vi "Configure Glitch Trigger Source.vi"(0 "VISA resource name":refnum<visa-resource-name>, 5 "Trigger Source (0: Channel 1)":u16(ring) items=["Channel 1", "Channel 2", "Channel 3", "Channel 4", "DIG 0", "DIG 1", "DIG 2", "DIG 3", "DIG 4", "DIG 5", "DIG 6", "DIG 7", "DIG 8", "DIG 9", "DIG 10", "DIG 11", "DIG 12", "DIG 13", "DIG 14", "DIG 15", "External"], 7 "Trigger Level (0.0)":dbl, 9 "Glitch Condition (0: Less Than)":u16(ring) items=["Less Than", "Greater Than", "Range"], 11 "error in (no error)":errorcluster, 12 "Glitch Polarity (0: Positive)":u16(ring) items=["Positive", "Negative"], 13 "Maximum (2)":dbl=2.0, 14 "Minimum (1)":dbl=1.0) -> (4 "VISA resource name out":refnum<visa-resource-name>, 15 "error out":errorcluster)   [LabVIEW 2017, in "Agilent 6000 Series.lvlib"]
doc: "This VI configures the glitch trigger. You specify the condition with the Glitch Condition property and polarity of the pulse with the Glitch Polarity parameter. The trigger does not actually occur until the edge of a pulse that corresponds to the Glitch Width and Glitch Polarity crosses the threshold you specify in the Trigger Level parameter."
uses:
  <instrlib>/Agilent 6000 Series/Agilent 6000 Series.lvlib
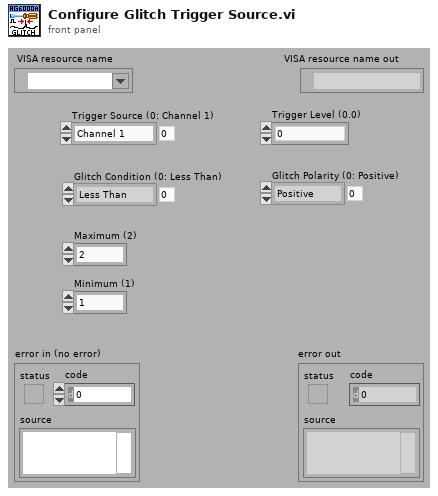
[diagram p1: front panel]
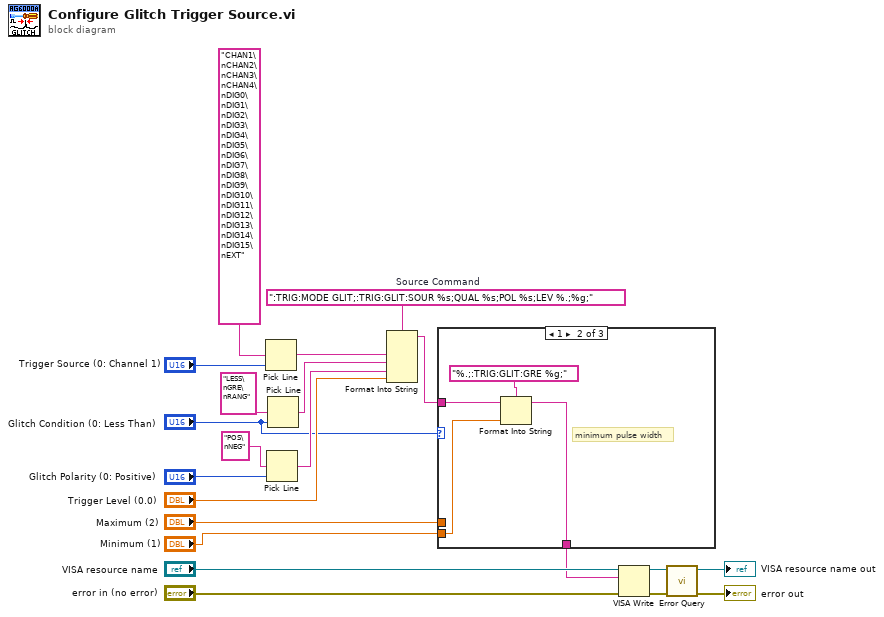
[diagram p0: block diagram]
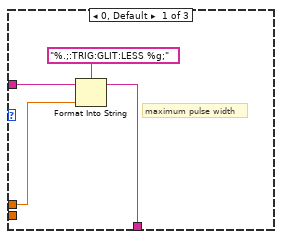
[diagram p2: hidden frame]
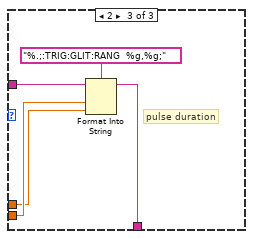
[diagram p3: hidden frame]
diagram:
  w15 = ":TRIG:MODE GLIT;:TRIG:GLIT:SOUR %s;QUAL %s;POL %s;LEV %.;%g;"  # Source Command
  n1 = Pick Line(multi-line string="CHAN1\nCHAN2\nCHAN3\nCHAN4\nDIG0\nDIG1\nDIG2\nDIG3\nDIG4\nDIG5\nDIG6\nDIG7\nDIG8\nDIG9\nDIG10\nDIG11\nDIG12\nDIG13\nDIG14\nDIG15\nEXT", line index="Trigger Source (0: Channel 1)") -> (output string=w14:string)  [unwired: 1 in]
  n2 = Pick Line(multi-line string="POS\nNEG", line index="Glitch Polarity (0: Positive)") -> (output string=w8:string)  [unwired: 1 in]
  n3 = Pick Line(multi-line string="LESS\nGRE\nRANG", line index="Glitch Condition (0: Less Than)") -> (output string=w11:string)  [unwired: 1 in]
  n4 = Format Into String(format string=w15, w14, w11, w8, "Trigger Level (0.0)") -> (resulting string=w4:string)  [unwired: 2 in, 1 out]
  n5 = case shown="1" "Glitch Condition (0: Less Than)" {
    tunnel: "Maximum (2)" -> [w24 _ w30]
    tunnel: w4 -> [w23 w28 w33]
    tunnel: [w22 w26 w31] -> w3
    tunnel: "Minimum (1)" -> [_ w27 w32]
    frame 0, Default {
      # "maximum pulse width"
      n6 = Format Into String(format string="%.;:TRIG:GLIT:LESS %g;", initial string=w23, w24) -> (resulting string=w22:string)  [unwired: 1 in, 1 out]
    }
    frame 1 {
      # "minimum pulse width"
      n7 = Format Into String(format string="%.;:TRIG:GLIT:GRE %g;", initial string=w28, w27) -> (resulting string=w26:string)  [unwired: 1 in, 1 out]
    }
    frame 2 {
      # "pulse duration"
      n8 = Format Into String(format string="%.;:TRIG:GLIT:RANG  %g,%g;", initial string=w33, w32, w30) -> (resulting string=w31:string)  [unwired: 1 in, 1 out]
    }
  }
  n9 = VISA Write(VISA resource name="VISA resource name", write buffer=w3, error in (no error)="error in (no error)") -> (VISA resource name out=w17:refnum<visa-resource-name>, error out=w16:errorcluster)  [unwired: 1 out]
  n10 = call <instrlib>:"Error Query.vi"("error in (no error)"=w16, "VISA resource name"=w17) -> ("error out"=→"error out":errorcluster, "VISA resource name out"=→"VISA resource name out":refnum<visa-resource-name>)  [unwired: 6 in, 2 out]
